vi "Load-Save Hardware Config.vi"(6 "Backup file path":path, 7 "Standalone ?":bool, 8 "error in":errorcluster, 9 "Hardware Configuration I/P":T1={"Dev. PC"=FALSE, "Swap XY on stage"=FALSE, "No of AOD"=0, "MC Supported"=FALSE, "Axial MC"=FALSE, "Computer MAC address"="", "Externalise Triggers"=FALSE, "Trigger HW config"={"Available Device List"=0, "Device Address"=""}, "DAQmx Chan"={"Pockels AO"="", "Hard shutter AO"="", "PMT AOs"="", "Galvo AOs"="", "Power meter AI"=""}, "XYZ Stage Control Config"=enum."None", "XY stage available"=FALSE, "XY Comms Config Cluster"={"Name"="COM7", "Device Address"="", "Port "=0, "Baudrate"=0, "Comms Type"=enum."GPIB-IEEE488"}, "Y stage available"=FALSE, "Y Comms Config Cluster"={"Name"="", "Device Address"="", "Port "=0, "Baudrate"=0, "Comms Type"=enum."GPIB-IEEE488"}, "Z stage available"=FALSE, "Z Comms Config Cluster "={"Name"="", "Device Address"="", "Port "=0, "Baudrate"=0, "Comms Type"=enum."GPIB-IEEE488"}, "Encoder available"=FALSE, "Encoder"={"IP address"="224.0.1.103", "Port"=7000, "Wheel radius (cm)"=16.0, "Encoder Trigger"=""}, "VidRec available"=FALSE, "Cam VidRec"={"DO flag-Video record"="", "DO flag-Trial start"=""}, "Laser Power Control HW config"={"Laser Power Control"="", "Laser Power Modulation Control"=enum."NI"}, "Laser 1 available"=FALSE, "Laser 1 config cluster"={"COM port"="COM7", "Baud Rate"=0, "Type"=""}, "Prechirper 1 available"=FALSE, "Prechirper 1 config cluster"={"Type"="", "Baud Rate"=0, "COM port"="COM7"}, "Control system.FPGA available?"=FALSE, "Control Sys. HW config"={"Control system.FPGA Type"=enum."Virtex 5", "Control system.Network adapter name"="", "Control system.MAC address"="", "Control system.Ethernet Port"=0, "Control system.Ethernet Port Opened"=FALSE}, "DAQ FPGA HW Config"={"FGPA Ref"=refnum, "Target"="RIO0", "input card type"=enum."AC Card"}, "PMT Control Voltage Limits"={"Lower Limit"=0.0, "Upper Limit"=0.0}} {"Encoder"."Wheel radius (cm)" format="%#_13g"}, 11 "Function":T18=enum."Load from file") -> (0 "error out":errorcluster, 1 "Hardware Configuration O/P":T1={"Dev. PC"=FALSE, "Swap XY on stage"=FALSE, "No of AOD"=0, "MC Supported"=FALSE, "Axial MC"=FALSE, "Computer MAC address"="", "Externalise Triggers"=FALSE, "Trigger HW config"={"Available Device List"=0, "Device Address"=""}, "DAQmx Chan"={"Pockels AO"="", "Hard shutter AO"="", "PMT AOs"="", "Galvo AOs"="", "Power meter AI"=""}, "XYZ Stage Control Config"=enum."None", "XY stage available"=FALSE, "XY Comms Config Cluster"={"Name"="COM7", "Device Address"="", "Port "=0, "Baudrate"=0, "Comms Type"=enum."GPIB-IEEE488"}, "Y stage available"=FALSE, "Y Comms Config Cluster"={"Name"="", "Device Address"="", "Port "=0, "Baudrate"=0, "Comms Type"=enum."GPIB-IEEE488"}, "Z stage available"=FALSE, "Z Comms Config Cluster "={"Name"="", "Device Address"="", "Port "=0, "Baudrate"=0, "Comms Type"=enum."GPIB-IEEE488"}, "Encoder available"=FALSE, "Encoder"={"IP address"="224.0.1.103", "Port"=7000, "Wheel radius (cm)"=16.0, "Encoder Trigger"=""}, "VidRec available"=FALSE, "Cam VidRec"={"DO flag-Video record"="", "DO flag-Trial start"=""}, "Laser Power Control HW config"={"Laser Power Control"="", "Laser Power Modulation Control"=enum."NI"}, "Laser 1 available"=FALSE, "Laser 1 config cluster"={"COM port"="COM7", "Baud Rate"=0, "Type"=""}, "Prechirper 1 available"=FALSE, "Prechirper 1 config cluster"={"Type"="", "Baud Rate"=0, "COM port"="COM7"}, "Control system.FPGA available?"=FALSE, "Control Sys. HW config"={"Control system.FPGA Type"=enum."Virtex 5", "Control system.Network adapter name"="", "Control system.MAC address"="", "Control system.Ethernet Port"=0, "Control system.Ethernet Port Opened"=FALSE}, "DAQ FPGA HW Config"={"FGPA Ref"=refnum, "Target"="RIO0", "input card type"=enum."AC Card"}, "PMT Control Voltage Limits"={"Lower Limit"=0.0, "Upper Limit"=0.0}} {"Encoder"."Wheel radius (cm)" format="%#_13g"})   [LabVIEW 2020]
uses:
  <vilib>/Utility/config.llb/NI_LVConfig.lvlib
  Typedefs/Which path.ctl
  <vilib>/userDefined/High Color/nirio_resource_hc.ctl
  Typedefs/DAQmx physical channels cluster.ctl
  Typedefs/Save-Load enum.ctl
  Typedefs/FPGA input type AC-DC.ctl
  Typedefs/Encoder config cluster.ctl
  Typedefs/Cam VidRec HW config setup cluster.ctl
  Typedefs/Control Sys HW config cluster.ctl
  Typedefs/Triggers HW config.ctl
  Typedefs/Laser 1 config cluster.ctl
  Typedefs/PreChirper 1 config cluster.ctl
  Typedefs/Laser Power Control HW config.ctl
  Typedefs/Hardware Configuration settings.ctl
  RIG-SPECIFIC FILES/FPGA Refs/FPGA Ref.ctl
  Typedefs/DAQ FPGA HW config cluster.ctl
  Typedefs/PMT Control Voltage limits.ctl
  Peripherals Control/XYZ Stage/Control/typedefs/XYZControlConfig.ctl
  Typedefs/Comms Type.ctl
  Typedefs/Peripherals comms config cluster.ctl
panel:
  # "<--- The \"PMT AOs\" DAQmx string will always contain\n                       2 channels is this format: PXI1Slot4/ao2:3"
  # "(make , model etc)"
  # "(COM Port / IP Address / service address etc.)"
  # "(Port for ethernet / channel for BT)"
  # "(make , model etc)"
  # "(COM Port / IP Address / service address etc.)"
  # "(Port for ethernet / channel for BT)"
  # "(make , model etc)"
  # "(COM Port / IP Address / service address etc.)"
  # "(Port for ethernet / channel for BT)"
  # "(make , model etc)"
  # "(COM Port / IP Address / service address etc.)"
  # "(Port for ethernet / channel for BT)"
  # "(make , model etc)"
  # "(COM Port / IP Address / service address etc.)"
  # "(Port for ethernet / channel for BT)"
  # "(make , model etc)"
  # "(COM Port / IP Address / service address etc.)"
  # "(Port for ethernet / channel for BT)"
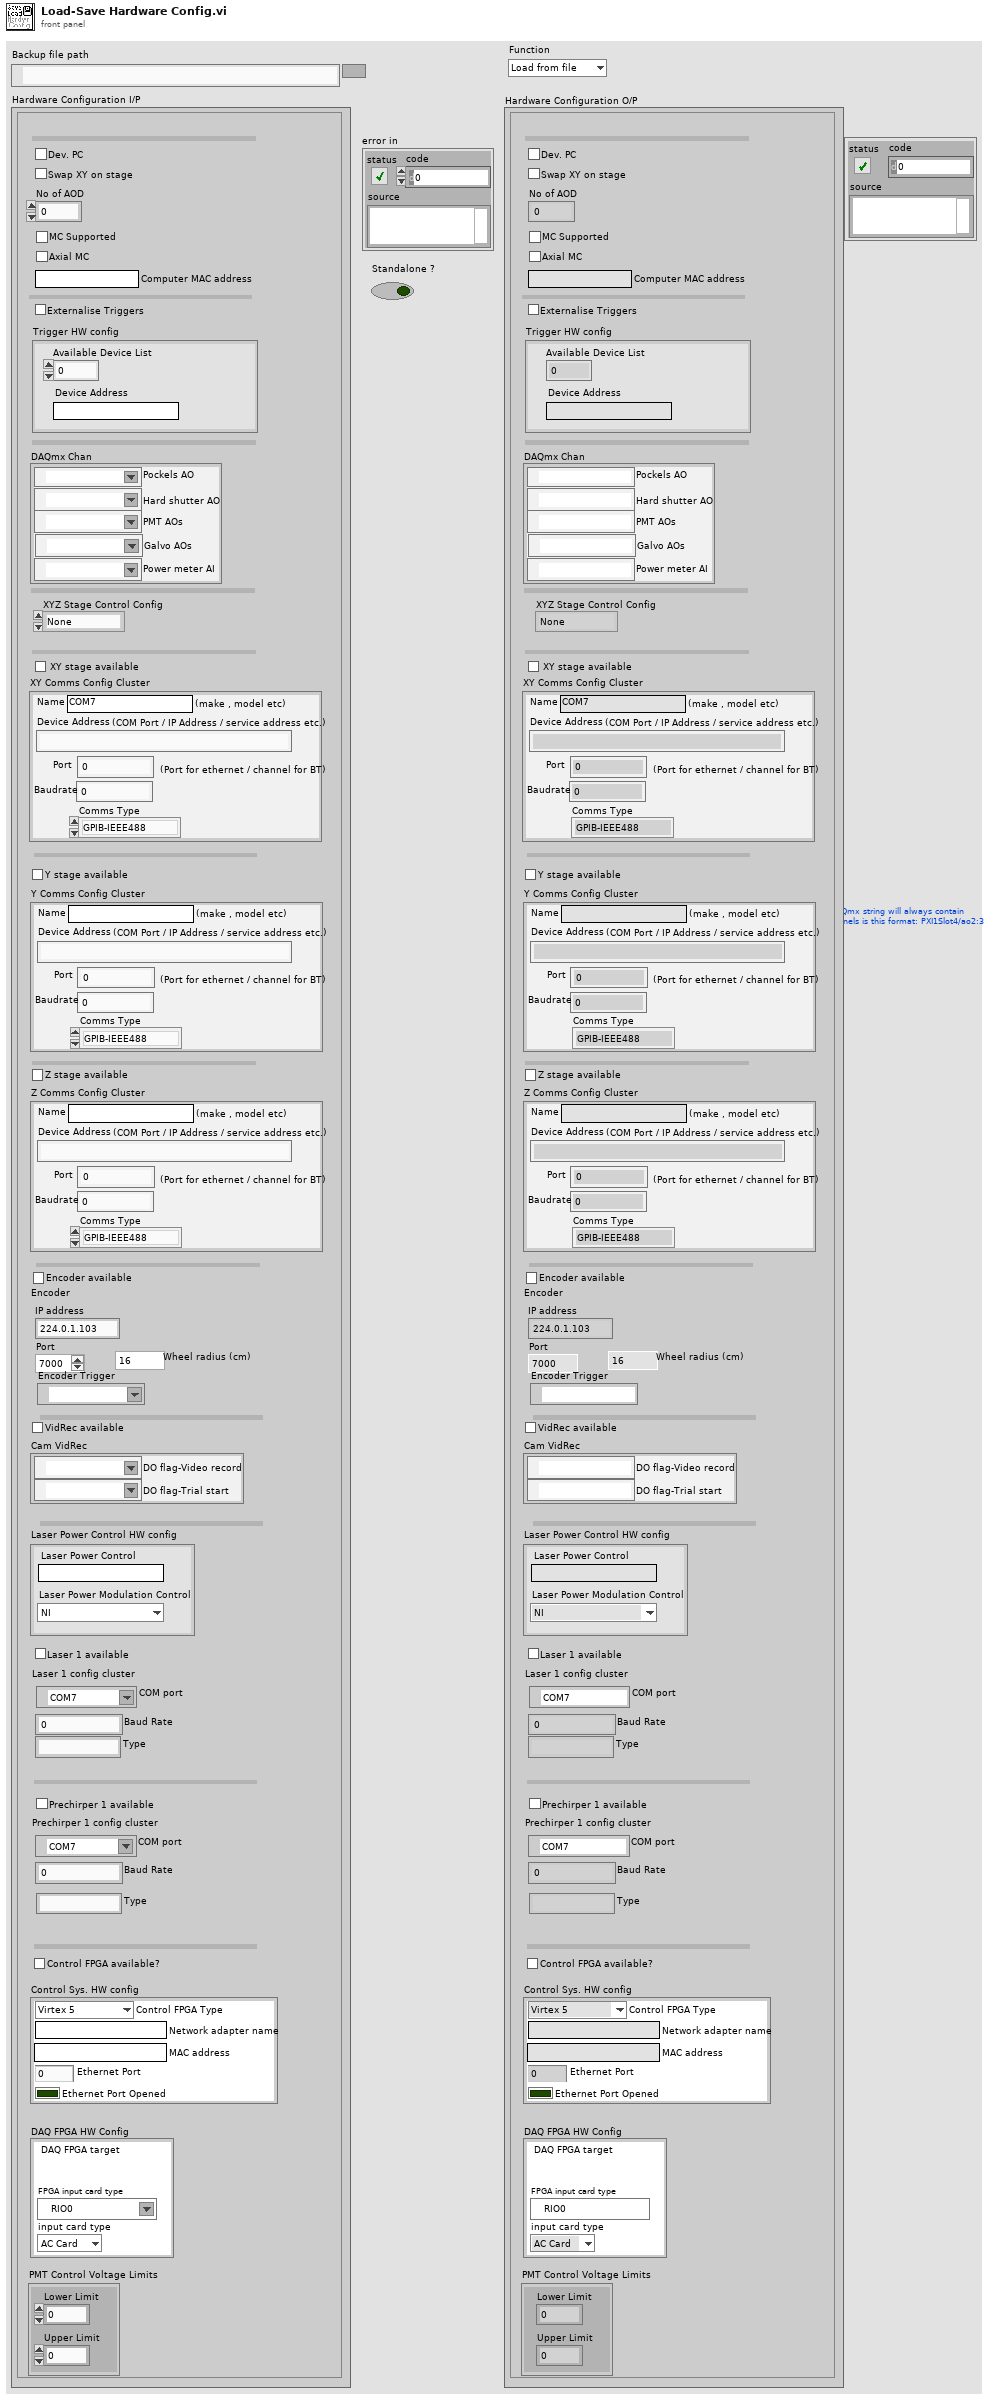
[diagram p1: front panel]
types:
  T1 = typedef "Hardware Configuration settings.ctl" = cluster{"Dev. PC":bool, "Swap XY on stage":bool, "No of AOD":u8, "MC Supported":bool, "Axial MC":bool, "Computer MAC address":string, "Externalise Triggers":bool, "Trigger HW config":T2, "DAQmx Chan":T3, "XYZ Stage Control Config":T4, "XY stage available":bool, "XY Comms Config Cluster":T5, "Y stage available":bool, "Y Comms Config Cluster":T5, "Z stage available":bool, "Z Comms Config Cluster ":T5, "Encoder available":bool, "Encoder":T7, "VidRec available":bool, "Cam VidRec":T8, "Laser Power Control HW config":T9, "Laser 1 available":bool, "Laser 1 config cluster":T10, "Prechirper 1 available":bool, "Prechirper 1 config cluster":T11, "Control system.FPGA available?":bool, "Control Sys. HW config":T12, "DAQ FPGA HW Config":T13, "PMT Control Voltage Limits":T17}
  T2 = typedef "Triggers HW config.ctl" = cluster{"Available Device List":i32, "Device Address":string}
  T3 = typedef "DAQmx physical channels cluster.ctl" = cluster{"Pockels AO":tag, "Hard shutter AO":tag, "PMT AOs":tag, "Galvo AOs":tag, "Power meter AI":tag}
  T4 = typedef "XYZControlConfig.ctl" = enum16{"None", "XYZ", "XY-Z", "X-Y-Z", "Z"}
  T5 = typedef "Peripherals comms config cluster.ctl" = cluster{"Name":string, "Device Address":string, "Port ":u16, "Baudrate":i32, "Comms Type":T6}
  T6 = typedef "Comms Type.ctl" = enum16{"GPIB-IEEE488", "Serial-RS232", "Serial-RS485", "Serial-RS422", "Serial-USB", "Ethernet-TCP/IP", "Ethernet-UDP"}
  T7 = typedef "Encoder config cluster.ctl" = cluster{"IP address":string, "Port":u16, "Wheel radius (cm)":dbl, "Encoder Trigger":tag}
  T8 = typedef "Cam VidRec HW config setup cluster.ctl" = cluster{"DO flag-Video record":tag, "DO flag-Trial start":tag}
  T9 = typedef "Laser Power Control HW config.ctl" = cluster{"Laser Power Control":string, "Laser Power Modulation Control":enum16{"NI", "FPGA"}}
  T10 = typedef "Laser 1 config cluster.ctl" = cluster{"COM port":refnum<visa-resource-name>, "Baud Rate":i32, "Type":string}
  T11 = typedef "PreChirper 1 config cluster.ctl" = cluster{"Type":string, "Baud Rate":i32, "COM port":refnum<visa-resource-name>}
  T12 = typedef "Control Sys HW config cluster.ctl" = cluster{"Control system.FPGA Type":enum16{"Virtex 5", "Virtex 7"}, "Control system.Network adapter name":string, "Control system.MAC address":string, "Control system.Ethernet Port":u32, "Control system.Ethernet Port Opened":bool}
  T13 = typedef "DAQ FPGA HW config cluster.ctl" = cluster{"FGPA Ref":T14, "Target":T15, "input card type":T16}
  T14 = typedef "FPGA Ref.ctl" = refnum<k20>
  T15 = typedef "nirio_resource_hc.ctl" = tag
  T16 = typedef "FPGA input type AC-DC.ctl" = enum16{"AC Card", "DC Card"}
  T17 = typedef "PMT Control Voltage limits.ctl" = cluster{"Lower Limit":dbl, "Upper Limit":dbl}
  T18 = typedef "Save-Load enum.ctl" = enum16{"Save to file", "Load from file", "Compare from file", "Save Backup"}
  T19 = typedef "Which path.ctl" = enum16{"Configuration Files", "Calibration Files", "Images", "Setup.ini", "Loaded User profile.ini", "User's-Previous session.ini", "New user profile.ini", "Selected User profile.ini", "User profiles folder", "Power meter scaling.txt", "FOV Cal.ini", "Calibration.ini"}
  T20 = typedef "NI_LVConfig.lvlib/Config Data RefNum.ctl" = refnum<k1>
  T21 = typedef "Ini file interface (String).ctl" = cluster{"key":string, "Save?":bool, "Default":string}[]
  T22 = typedef "Ini file interface (DBL).ctl" = cluster{"key":string, "Save?":bool, "Default":dbl}[]
  T23 = typedef "Ini file interface (Boolean).ctl" = cluster{"key":string, "Save?":bool, "Default":bool}[]
  T24 = cluster{"key":string, "Save?":bool, "Default":dbl}
  T25 = cluster{"key":string, "Save?":bool, "Default":dbl}[]
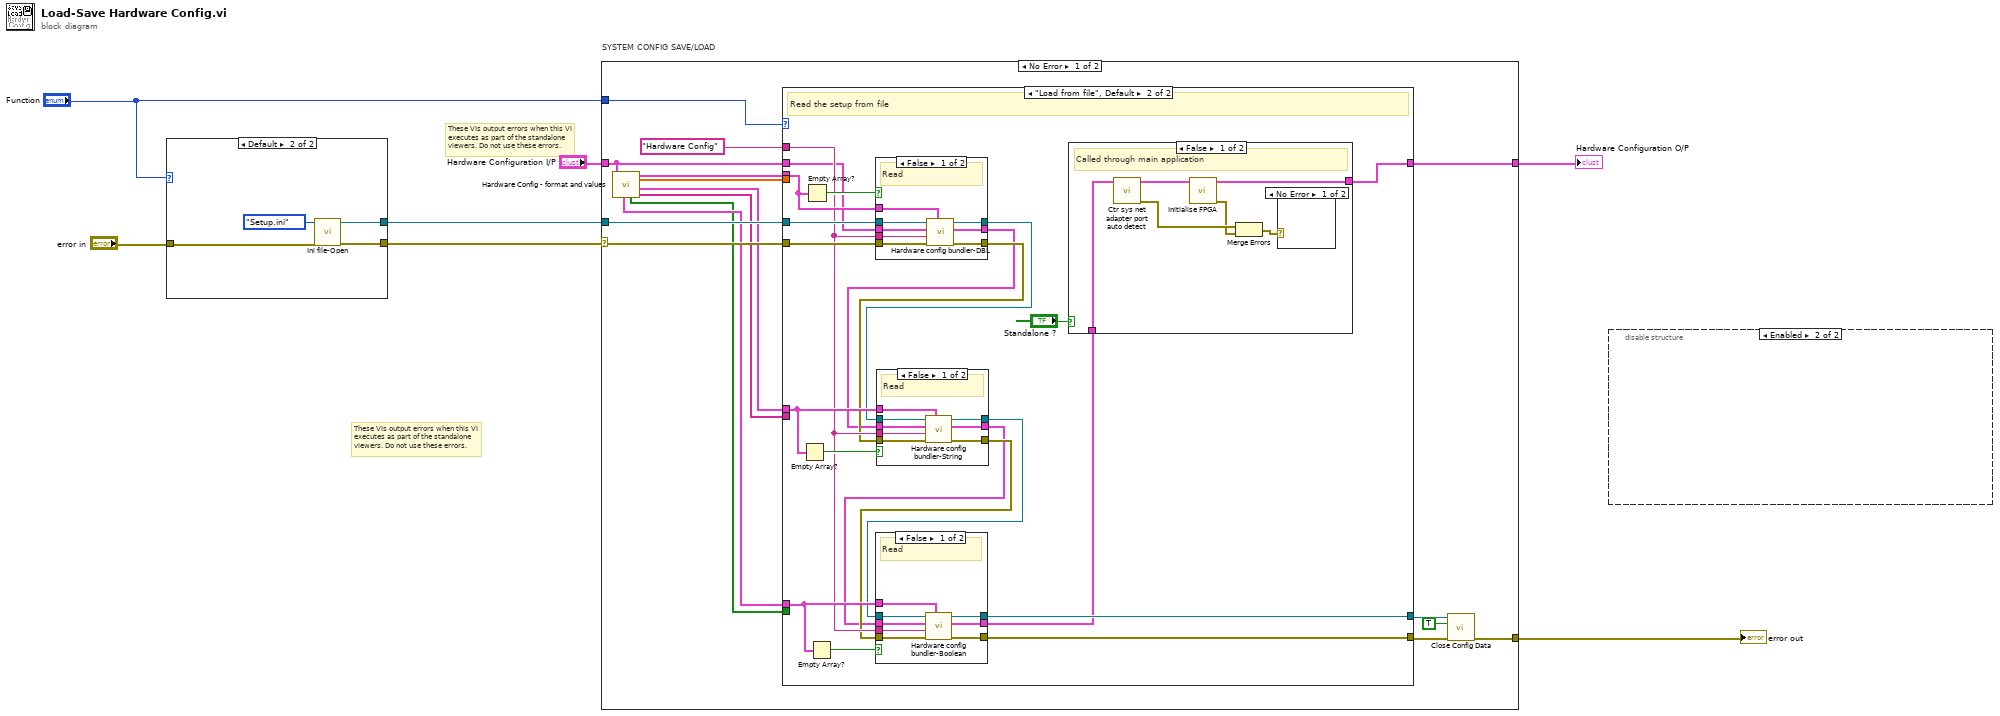
[diagram p0: block diagram]
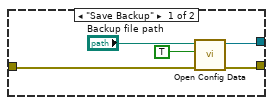
[diagram p2: hidden frame]
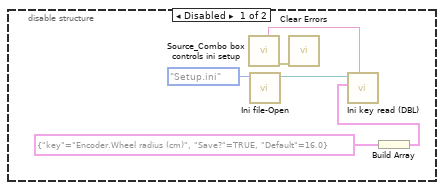
[diagram p3: hidden frame]
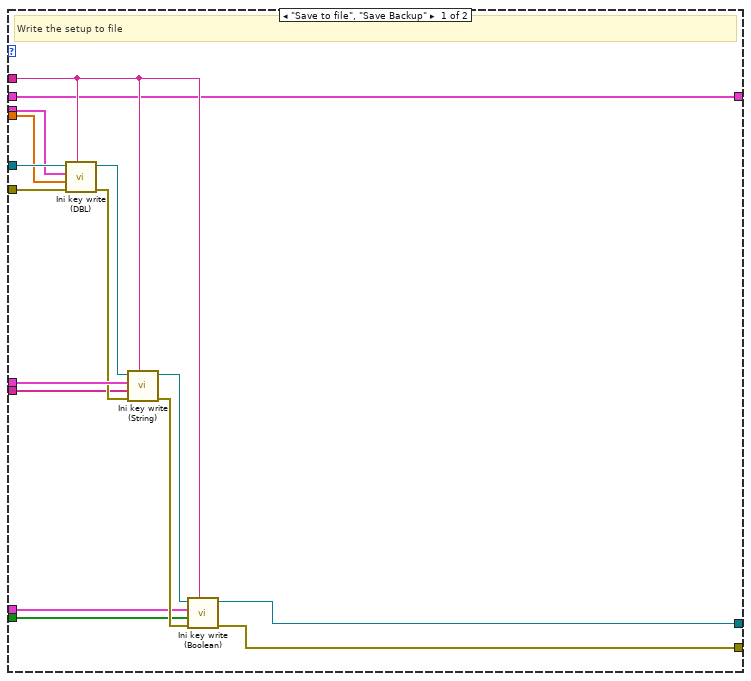
[diagram p4: hidden frame]
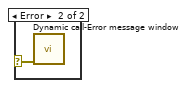
[diagram p5: hidden frame]
diagram:
  # "These VIs output errors when this VI executes as part of the standalone viewers. Do not use these errors."
  # "These VIs output errors when this VI executes as part of the standalone viewers. Do not use these errors."
  n1 = case shown="Default" "Function" {
    tunnel: [w9 w15] -> w3
    tunnel: [w10 w14] -> w2
    tunnel: "error in" -> [w11 w13]
    frame "Save Backup" {
      n2 = call <vilib>:"Open Config Data.vi"("error in (no error)"=w11, "create file if necessary (T)"=TRUE ("create file if necessary"), "configuration file path"="Backup file path") -> ("error out"=w9:errorcluster, "refnum"=w10:T20)  [unwired: 6 in, 1 out]
    }
    frame Default {
      n3 = call "Ini file-Open.vi"("Error In"=w13, "Which file?"=Which_path."Setup.ini") -> ("error out"=w15:errorcluster, "User profile ini file ref"=w14:T20)  [unwired: 6 in, 2 out]
    }
  }
  n4 = case "SYSTEM CONFIG SAVE/LOAD" shown="No Error" w3 {
    selector: w3 -> [w28 w112]
    tunnel: [w26 w112] -> w7
    tunnel: "Hardware Configuration I/P" -> [w21 w111]
    tunnel: [w30 w111] -> w5
    tunnel: "Function" -> [w29 _]
    tunnel: w2 -> [w27 _]
    frame No Error {
      n5 = call "Hardware Config - format and values.vi"("Hardware Configuration"=w21) -> (0:"String"=w19:string[], 1:"String"=w20:T21, 2:"Numeric"=w22:dbl[], 3:"Numeric"=w23:T22, 4:"Boolean"=w17:bool[], 6:"Boolean"=w18:T23)  [unwired: 5 in]
      n6 = case shown="\"Load from file\", Default" w29 {
        tunnel: [w35 w64] -> w25
        tunnel: [w34 w65] -> w31
        tunnel: w28 -> [w47 w66]
        tunnel: w27 -> [w48 w69]
        tunnel: "Hardware Config" -> [w37 w59]
        tunnel: w23 -> [w45 w68]
        tunnel: w22 -> [w46 _]
        tunnel: w17 -> [w36 _]
        tunnel: w18 -> [w38 w63]
        tunnel: w19 -> [w41 _]
        tunnel: w20 -> [w44 w60]
        tunnel: [w33 w50] -> w30
        tunnel: w21 -> [w33 w54]
        frame "Save to file", "Save Backup" {
          # "Write the setup to file"
          n7 = call "Ini key write (DBL).vi"("Section"=w37, "error in (no error)"=w47, "Values (DBL)"=w46, "Ini file interface"=w45, "Ini file refnum in"=w48) -> ("error out"=w42:errorcluster, "Ini file refnum out"=w43:T20)  [unwired: 5 in]
          n8 = call "Ini key write (String).vi"("Section"=w37, "error in (no error)"=w42, "Values (String)"=w41, "Ini file interface"=w44, "Ini file refnum in"=w43) -> ("error out"=w39:errorcluster, "Ini file refnum out"=w40:T20)  [unwired: 5 in]
          n9 = call "Ini key write (Boolean).vi"("Section"=w37, "error in (no error)"=w39, "Values (Boolean)"=w36, "Ini file interface"=w38, "Ini file refnum in"=w40) -> ("error out"=w35:errorcluster, "Ini file refnum out"=w34:T20)  [unwired: 5 in]
        }
        frame "Load from file", Default {
          # "Read the setup from file"
          n10 = Empty Array?(array=w60) -> (empty?=w61:bool)
          n11 = Empty Array?(array=w68) -> (empty?=w67:bool)
          n12 = Empty Array?(array=w63) -> (empty?=w62:bool)
          n13 = case shown="False" w67 {
            tunnel: w69 -> [w107 w110]
            tunnel: [w106 w110] -> w55
            tunnel: [w105 w109] -> w56
            tunnel: w66 -> [w104 w109]
            tunnel: w59 -> [w102 _]
            tunnel: w68 -> [w103 _]
            tunnel: w54 -> [w100 w108]
            tunnel: [w101 w108] -> w53
            frame False {
              # "Read"
              n14 = call "Hardware config bundler-DBL.vi"("Keys setup.DBL"=w103, "error in (no error)"=w104, "Section name"=w102, "Hardware Configuration"=w100, "Refnum in"=w107) -> ("error out"=w105:errorcluster, "output cluster"=w101:T1, "Refnum out"=w106:T20)  [unwired: 4 in]
            }
            frame True {
              # "No parametersof such type"
            }
          }
          n15 = case shown="False" w61 {
            tunnel: [w82 w88] -> w58
            tunnel: [w81 w87] -> w57
            tunnel: w60 -> [w84 _]
            tunnel: w55 -> [w85 w88]
            tunnel: w56 -> [w80 w87]
            tunnel: w59 -> [w83 _]
            tunnel: w53 -> [w79 w86]
            tunnel: [w78 w86] -> w52
            frame False {
              # "Read"
              n16 = call "Hardware config bundler-String.vi"("Keys setup.String"=w84, "error in (no error)"=w80, "Section name"=w83, "Hardware Configuration I/P"=w79, "Refnum in"=w85) -> ("error out"=w81:errorcluster, "Hardware Configuration O/P"=w78:T1, "Refnum out"=w82:T20)  [unwired: 4 in]
            }
            frame True {
              # "No parametersof such type"
            }
          }
          n17 = case shown="False" w62 {
            tunnel: [w95 w99] -> w65
            tunnel: [w94 w98] -> w64
            tunnel: w63 -> [w91 _]
            tunnel: w58 -> [w96 w99]
            tunnel: w57 -> [w93 w98]
            tunnel: w59 -> [w92 _]
            tunnel: w52 -> [w89 w97]
            tunnel: [w90 w97] -> w51
            frame False {
              # "Read"
              n18 = call "Hardware config bundler-Boolean.vi"("Keys setup.Boolean"=w91, "error in (no error)"=w93, "Section name"=w92, "Hardware Configuration I/P"=w89, "Refnum in"=w96) -> ("error out"=w94:errorcluster, "Hardware Configuration O/P"=w90:T1, "Refnum out"=w95:T20)  [unwired: 4 in]
            }
            frame True {
              # "No parametersof such type"
            }
          }
          n19 = case shown="False" "Standalone ?" {
            tunnel: [w71 w77] -> w50
            tunnel: w51 -> [w70 w77]
            frame False {
              # "Called through main application"
              n20 = call "Ctr sys net adapter port auto detect.vi"("HW Config IN"=w70) -> ("error out"=w74:errorcluster, "HW config OUT"=w75:T1)  [unwired: 9 in]
              n21 = call "Initialise FPGA.vi"("Hardware Resources in"=w75) -> ("error out"=w73:errorcluster, "Hardware Resources out"=w71:T1)  [unwired: 9 in]
              n22 = Merge Errors(w74, w73) -> (w72:errorcluster)
              n23 = case shown="No Error" w72 {
                selector: w72 -> [_ w76]
                frame No Error {
                }
                frame Error {
                  n24 = call "Dynamic call-Error message window.vi"("error in (no error)"=w76) -> ()  [unwired: 10 in, 1 out]
                }
              }
            }
            frame True {
              # "Standalone viewer"
            }
          }
        }
      }
      n25 = call <vilib>:"Close Config Data.vi"("error in (no error)"=w25, "write file if changed (T)"=TRUE ("write configuration file? (F)"), "refnum"=w31) -> ("error out"=w26:errorcluster)  [unwired: 7 in, 1 out]
    }
    frame Error {
    }
  }
  "error out" <- w7
  "Hardware Configuration O/P" <- w5
  n26 = disable-structure shown="Enabled" {
    frame Disabled {
      n27 = call "Source_Combo box controls ini setup.vi"() -> ("error out"=w113:errorcluster, "Section name"=w114:string)  [unwired: 9 in, 1 out]
      n28 = call "Ini file-Open.vi"("Which file?"=Which_path."Setup.ini") -> ("User profile ini file ref"=w117:T20)  [unwired: 7 in, 3 out]
      n29 = call <vilib>:"Clear Errors.vi"("error in (no error)"=w113) -> ()  [unwired: 5 in, 2 out]
      n30 = Build Array(T24 {"key"="Encoder.Wheel radius (cm)", "Save?"=TRUE, "Default"=16.0}) -> (w115:T25)
      n31 = call "Ini key read (DBL).vi"("Section name"=w114, "Parameter names & setup"=w115, "Ini file refnum in"=w117) -> ()  [unwired: 6 in, 3 out]
    }
    frame Enabled {
    }
  }
